vi "Instantiate Module.vi"(8 "error in":errorcluster, 11 "Plugin in":refnum<class "Plugin.lvclass">) -> (0 "error out":errorcluster, 2 "Module Instance":refnum<class>, 3 "Plugin out":refnum<class "Plugin.lvclass">)   [LabVIEW 2020, in "Plugin.lvlib" / "Plugin.lvclass"]
uses:
  Plugin.lvclass
  Controller_Class/Plugin_Controller.lvclass
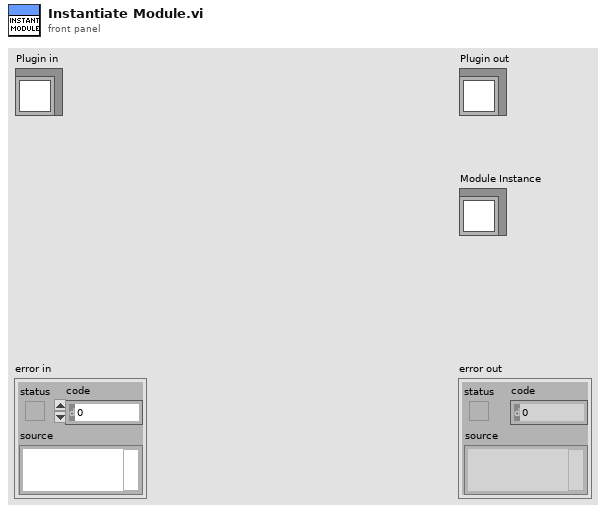
[diagram p1: front panel]
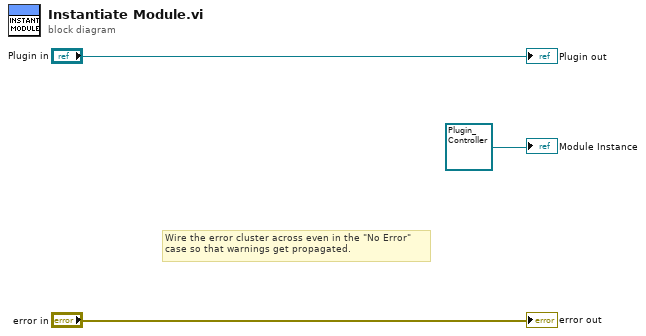
[diagram p0: block diagram]
diagram:
  # "Wire the error cluster across even in the \"No Error\"\ncase so that warnings get propagated."
  "error out" <- "error in"
  "Plugin out" <- "Plugin in"
  "Module Instance" <- refnum<class "Plugin_Controller.lvclass"> refnum ("Plugin.lvlib:Plugin_Controller.lvclass")
